vi "Easy_Keithley.vi"(10 "Final Thermocouple ID# (String)":string, 11 "First Thermocouple ID# (String)":string) -> (2 "Number of Thermocouples":dbl, 3 "concatenated string":string)   [LabVIEW 2015]
panel:
  out "Resulting string":string
  out "First Thermocouple ID# (int)":dbl
  out "Final Thermocouple ID# (int)":dbl
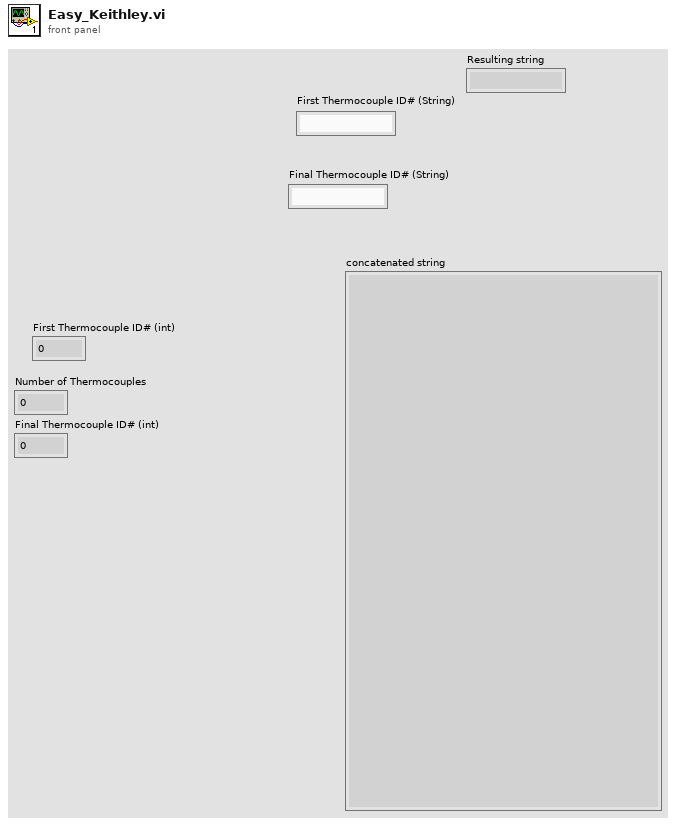
[diagram p1: front panel]
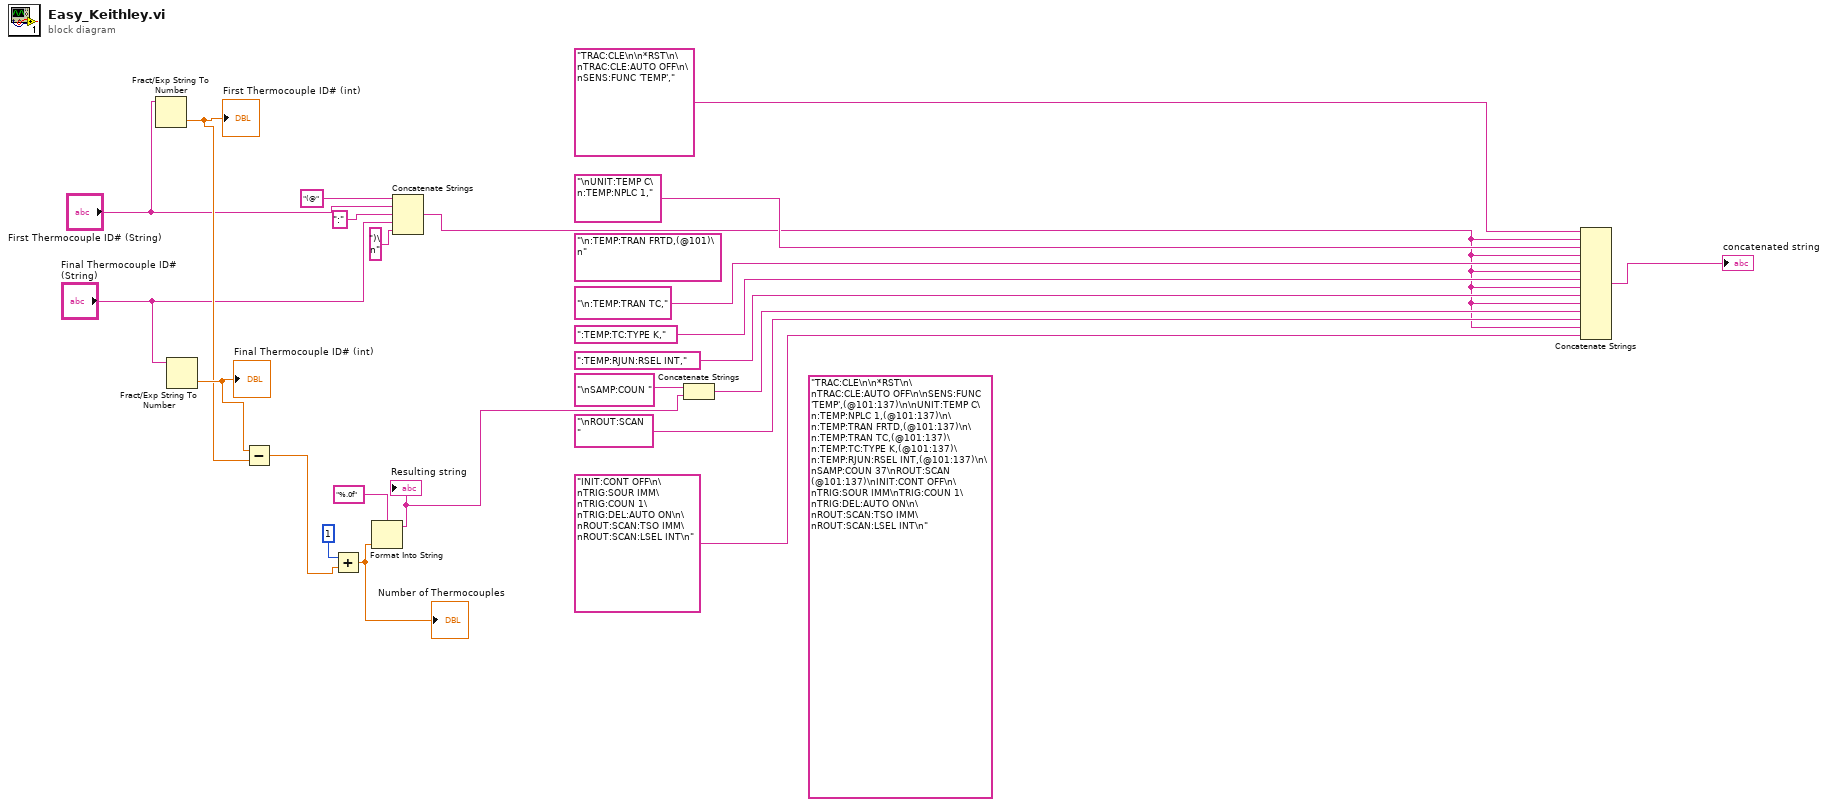
[diagram p0: block diagram]
diagram:
  (unwired) "TRAC:CLE\n\n*RST\n\nTRAC:CLE:AUTO OFF\n\nSENS:FUNC 'TEMP',(@101:137)\n\nUNIT:TEMP C\n:TEMP:NPLC 1,(@101:137)\n\n:TEMP:TRAN FRTD,(@101:137)\n\n:TEMP:TRAN TC,(@101:137)\n:TEMP:TC:TYPE K,(@101:137)\n:TEMP:RJUN:RSEL INT,(@101:137)\n\nSAMP:COUN 37\nROUT:SCAN  (@101:137)\nINIT:CONT OFF\n\nTRIG:SOUR IMM\nTRIG:COUN 1\nTRIG:DEL:AUTO ON\n\nROUT:SCAN:TSO IMM\nROUT:SCAN:LSEL INT\n"
  (unwired) "\n:TEMP:TRAN FRTD,(@101)\n"
  n1 = Fract/Exp String To Number(string="First Thermocouple ID# (String)") -> (number=w19:dbl)  [unwired: 3 in, 1 out]
  "First Thermocouple ID# (int)" <- w19
  n2 = Fract/Exp String To Number(string="Final Thermocouple ID# (String)") -> (number=w20:dbl)  [unwired: 3 in, 1 out]
  "Final Thermocouple ID# (int)" <- w20
  n3 = Subtract(x=w20, y=w19) -> (x-y=w16:dbl)
  n4 = Add(x=1, y=w16) -> (x+y=w1:dbl)
  "Number of Thermocouples" <- w1
  n5 = Format Into String(format string="%.0f", w1) -> (resulting string=w6:string)  [unwired: 2 in, 1 out]
  "Resulting string" <- w6
  n6 = Concatenate Strings("(@", "First Thermocouple ID# (String)", ":", "Final Thermocouple ID# (String)", ")\n") -> (w3:string)
  n7 = Concatenate Strings("\nSAMP:COUN ", w6) -> (w5:string)
  n8 = Concatenate Strings("TRAC:CLE\n\n*RST\n\nTRAC:CLE:AUTO OFF\n\nSENS:FUNC 'TEMP',", w3, "\nUNIT:TEMP C\n:TEMP:NPLC 1,", w3, "\n:TEMP:TRAN TC,", w3, ":TEMP:TC:TYPE K,", w3, ":TEMP:RJUN:RSEL INT,", w3, w5, "\nROUT:SCAN  ", w3, "INIT:CONT OFF\n\nTRIG:SOUR IMM\nTRIG:COUN 1\nTRIG:DEL:AUTO ON\n\nROUT:SCAN:TSO IMM\nROUT:SCAN:LSEL INT\n") -> (→"concatenated string":string)
